vi "Get Term Array.vi"(8 "error in (no error)":errorcluster, 11 "VI Refnum":refnum<vi>) -> (0 "error out":errorcluster, 2 "Terminals Array":T1[](array[typedef]), 3 "VI Reference out":refnum<vi>)   [LabVIEW 2012, in "Scripting Tools.lvlib" / "XNode Support.lvlib"]
doc: "Reads the connector pane of the vi with refnum <b>vi refnum</b> and returns an array that describes the connector pane terminals in a format that the GetTerms3 ability of an XNode can work with. This is useful for wrapping user supplied vi's in an XNode."
uses:
  XNode Support.lvlib
  <vilib>/XNodeSupport/XNodeTerm3.ctl
  <vilib>/XNodeSupport/XNodeString.ctl
  <vilib>/XNodeSupport/XNodeVariant.ctl
  <vilib>/XNodeSupport/XNodeRect32.ctl
  <vilib>/XNodeSupport/XNodeInt.ctl
  <vilib>/XNodeSupport/XNodeBool.ctl
  <vilib>/XNodeSupport/XNodeTermDirection.ctl
  <vilib>/XNodeSupport/NI_XNodeSupport.lvlib
  Scripting Tools.lvlib
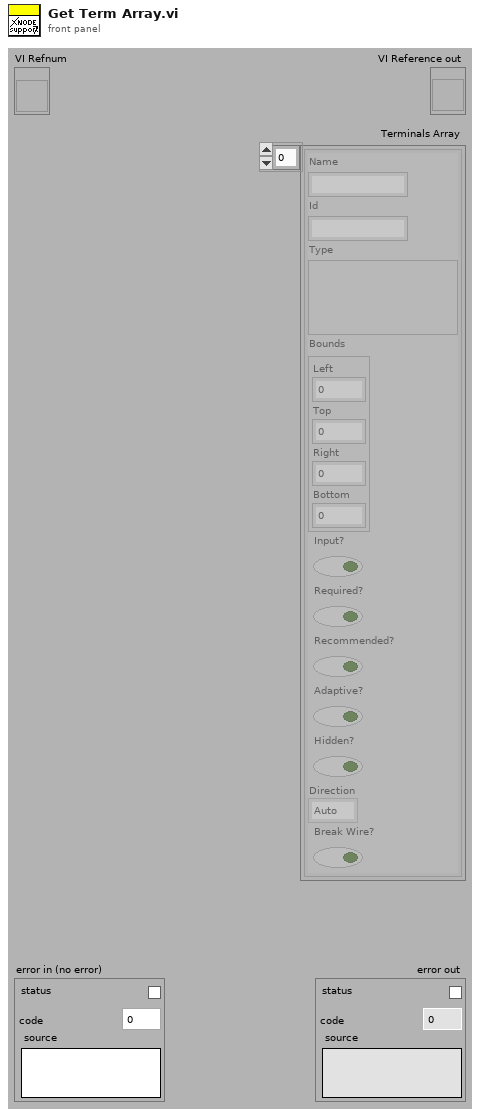
[diagram p1: front panel]
types:
  T1 = typedef "NI_XNodeSupport.lvlib/XNodeTerm3.ctl" = cluster{"Name":T2, "Id":T2, "Type":T3, "Bounds":T4, "Input?":T6, "Required?":T6, "Recommended?":T6, "Adaptive?":T6, "Hidden?":T6, "Direction":T7, "Break Wire?":T6}
  T2 = typedef "NI_XNodeSupport.lvlib/XNodeString.ctl" = string
  T3 = typedef "NI_XNodeSupport.lvlib/XNodeVariant.ctl" = variant
  T4 = typedef "NI_XNodeSupport.lvlib/XNodeRect32.ctl" = cluster{"Left":T5, "Top":T5, "Right":T5, "Bottom":T5}
  T5 = typedef "NI_XNodeSupport.lvlib/XNodeInt.ctl" = i32
  T6 = typedef "NI_XNodeSupport.lvlib/XNodeBool.ctl" = bool
  T7 = typedef "NI_XNodeSupport.lvlib/XNodeTermDirection.ctl" = enum32{"Auto", "Up", "Down", "Left", "Right", "Center"}
  T8 = typedef "LVRectTypeDef.ctl" = cluster{"Left":i16, "Top":i16, "Right":i16, "Bottom":i16}
  T9 = enum16{"Invalid Wire Rule", "Required", "Recommended", "Optional", "Dynamic Dispatch"}[]
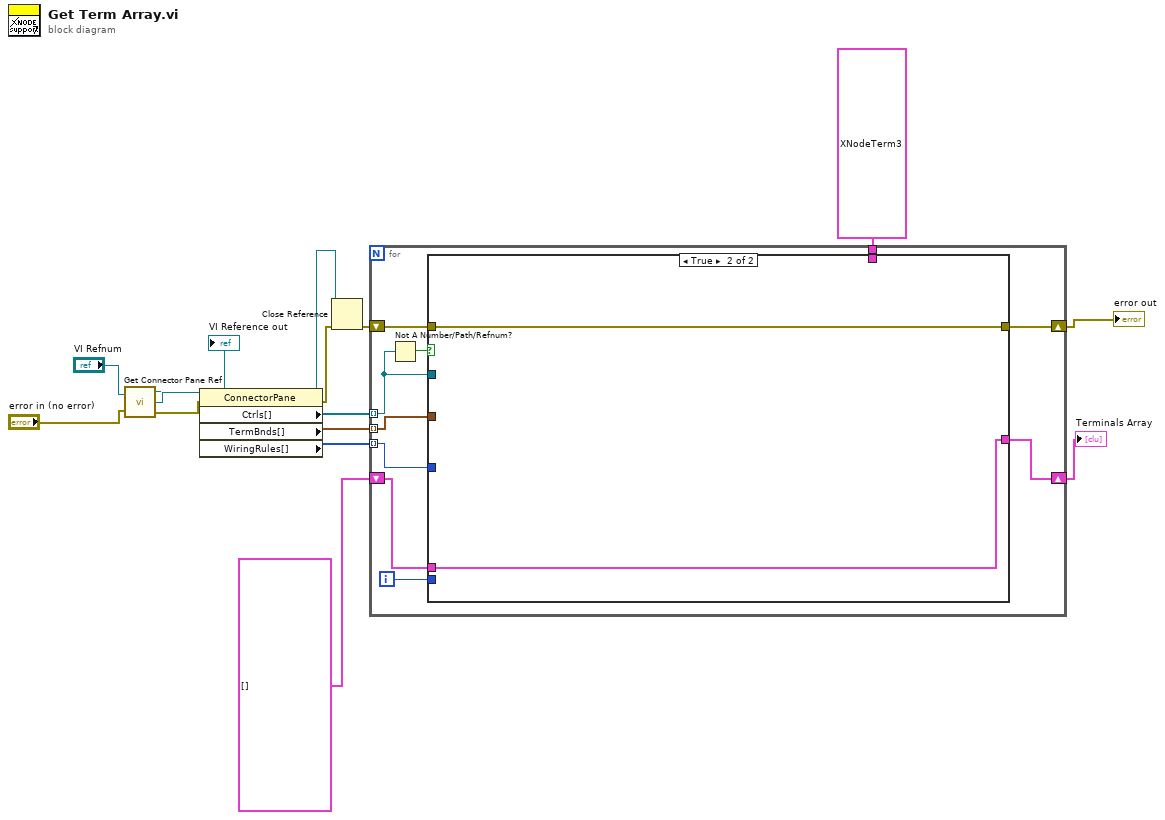
[diagram p0: block diagram]
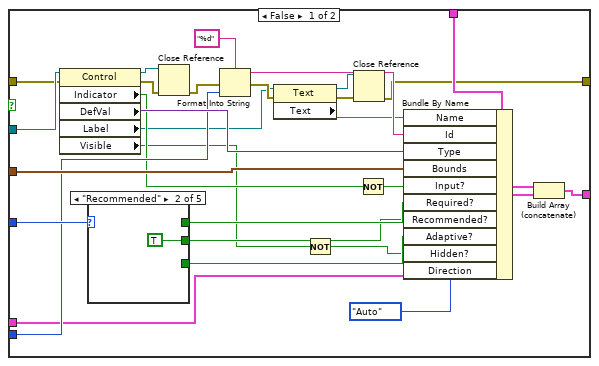
[diagram p2: hidden frame]
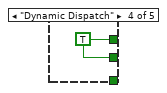
[diagram p5: hidden frame]
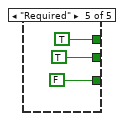
[diagram p6: hidden frame]
diagram:
  n1 = call "Get Connector Pane Ref.vi"("VI Reference"="VI Refnum", "error in (no error)"="error in (no error)") -> ("VI Reference out"=→"VI Reference out":refnum<vi>, "Connector Pane"=w13:refnum<vi>, "error out"=w12:errorcluster)
  n2 = property class="ConnectorPane"(reference=w13, error in=w12) -> (reference out=w6:refnum<vi>, error out=w8:errorcluster, "Ctrls[]"=w11:refnum<vi>[], "TermBnds[]"=w10:T8[], "WiringRules[]"=w9:T9)
  n3 = Close Reference(reference=w6, error in (no error)=w8) -> (error out=w7:errorcluster)
  n4 = for {
    tunnel: T1 {"Name"="Inputs", "Id"="", "Type"=variant, "Bounds"={"Left"=0, "Top"=0, "Right"=15, "Bottom"=0}, "Input?"=TRUE, "Required?"=TRUE, "Recommended?"=TRUE, "Adaptive?"=FALSE, "Hidden?"=FALSE, "Direction"=enum."Left", "Break Wire?"=FALSE} ("Term 3") -> [w25]
    tunnel: w11 -> [w17] mode=indexing
    tunnel: w10 -> [w24] mode=indexing
    tunnel: w9 -> [w23] mode=indexing
    shift-right: [w20] -> w2
    shift-left: w7 -> [w22]
    shift-right: [w19] -> w5
    shift-left: T1[] [] -> [w18]
    i -> [w21]
    n5 = Not A Number/Path/Refnum?(number/path/refnum=w17) -> (NaN/Path/Refnum?=w16:bool)
    n6 = case shown="True" w16 {
      tunnel: w25 -> [w54 _]
      tunnel: w24 -> [w53 _]
      tunnel: w23 -> [w52 _]
      tunnel: w17 -> [w47 _]
      tunnel: w22 -> [w46 w60]
      tunnel: w21 -> [w42 _]
      tunnel: [w30 w60] -> w20
      tunnel: [w27 w61] -> w19
      tunnel: w18 -> [w26 w61]
      frame False {
        n7 = property class="Control"(reference=w47, error in=w46) -> (reference out=w34:refnum<vi>, error out=w35:errorcluster, "Indicator"=w38:bool, "DefVal"=w44:variant, "Label"=w29:refnum<vi>, "Visible"=w37:bool)
        n8 = case shown="\"Recommended\"" w52 {
          tunnel: [_ _ _ w56 TRUE] -> w51
          tunnel: [_ TRUE _ w56 TRUE] -> w50
          tunnel: [_ _ _ _ FALSE] -> w49
          frame "Invalid Wire Rule", Default {
          }
          frame "Recommended" {
          }
          frame "Optional" {
          }
          frame "Dynamic Dispatch" {
            w56 = TRUE
          }
          frame "Required" {
          }
        }
        n9 = Close Reference(reference=w34, error in (no error)=w35) -> (error out=w33:errorcluster)
        n10 = Format Into String(format string="%d", error in=w33, w42) -> (resulting string=w41:string, error out=w40:errorcluster)  [unwired: 1 in]
        n11 = property class="Text"(reference=w29, error in=w40) -> (reference out=w31:refnum<vi>, error out=w32:errorcluster, "Text"=w39:string)
        n12 = Not(x=w37) -> (.not. x?=w36:bool)
        n13 = Close Reference(reference=w31, error in (no error)=w32) -> (error out=w30:errorcluster)
        n14 = Not(x=w38) -> (.not. x?=w45:bool)
        n15 = Bundle By Name(cluster=w54, "Name"=w39, "Id"=w41, "Type"=w44, "Bounds"=w53, "Input?"=w45, "Required?"=w51, "Recommended?"=w50, "Adaptive?"=w49, "Hidden?"=w36, "Direction"=XNodeTermDirection."Auto") -> (w28:T1)
        n16 = Build Array (concatenate)(w26, w28) -> (w27:T1[])
      }
      frame True {
      }
    }
  }
  "error out" <- w2
  "Terminals Array" <- w5
